vi "checkConnection.vi"(8 "error in (no error)":errorcluster, 11 "TCPClient in":refnum<class "TCPClient.lvclass">) -> (0 "error out":errorcluster, 3 "TCPClient out":refnum<class "TCPClient.lvclass">)   [LabVIEW 2016, in "TCPClient.lvclass"]
uses:
  TCPClient.lvclass
  TCPClient.lvclass/TCPClient.ctl
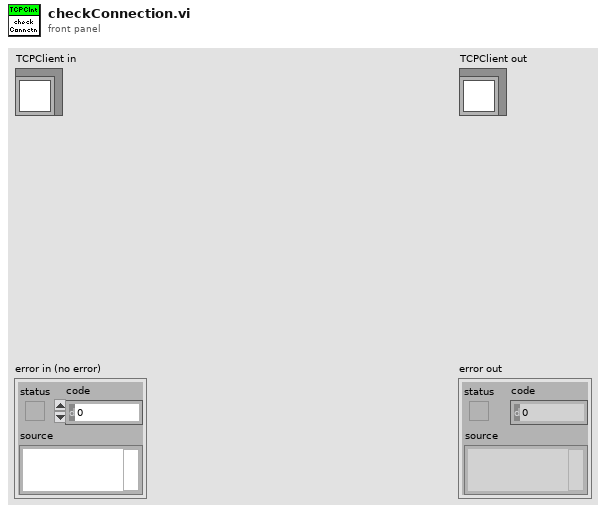
[diagram p1: front panel]
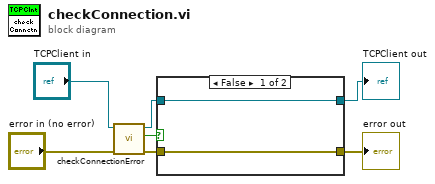
[diagram p0: block diagram]
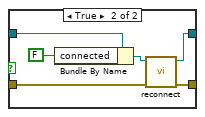
[diagram p2: hidden frame]
diagram:
  n1 = call "checkConnectionError.vi"("error in (no error)"="error in (no error)", "TCPClient in"="TCPClient in") -> ("error out"=w4:errorcluster, "ConnectionError?"=w3:bool, "TCPClient out"=w1:refnum<class "TCPClient.lvclass">)  [unwired: 7 in]
  n2 = case shown="False" w3 {
    tunnel: w1 -> [w9 w12]
    tunnel: w4 -> [w8 w15]
    tunnel: [w8 w14] -> w7
    tunnel: [w9 w13] -> w6
    frame False {
    }
    frame True {
      n3 = Bundle By Name(cluster=w12, "connected"=FALSE) -> (w11:refnum<class "TCPClient.lvclass">)
      n4 = call "reconnect.vi"("error in (no error)"=w15, "TCPClient in"=w11) -> ("error out"=w14:errorcluster, "TCPClient out"=w13:refnum<class "TCPClient.lvclass">)  [unwired: 8 in]
    }
  }
  "error out" <- w7
  "TCPClient out" <- w6
